vi "LabCode.vi"() -> ()   [LabVIEW 2020]
panel:
  in  "STOP":bool
  in  "GREEN":bool
  in  "YELLOW":bool
  in  "RED":bool
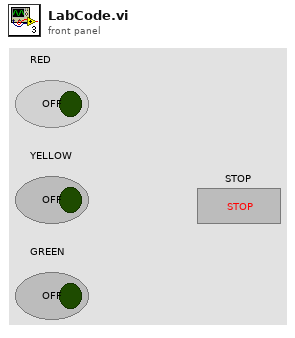
[diagram p1: front panel]
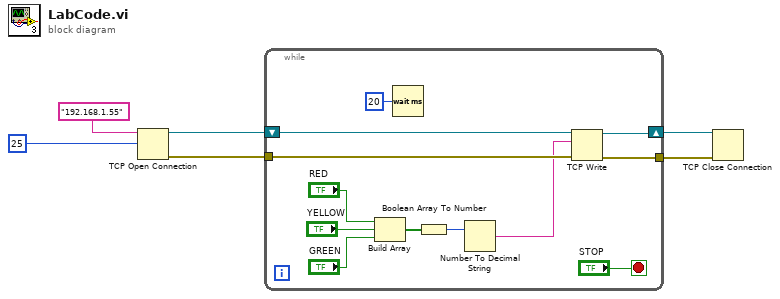
[diagram p0: block diagram]
diagram:
  n1 = TCP Open Connection(address="192.168.1.55", remote port or service name=u16 25) -> (connection ID=w4:refnum<k5>, error out=w3:errorcluster)  [unwired: 3 in]
  n2 = while {
    tunnel: w3 -> [w16]
    shift-right: [w15] -> w2
    shift-left: w4 -> [w17]
    tunnel: [w8] -> w1
    stop <- "STOP" stop-if-true
    n3 = Build Array("RED", "YELLOW", "GREEN") -> (w11:bool[])
    n4 = Wait (ms)(milliseconds to wait=u32 20) -> ()  [unwired: 1 out]
    n5 = Boolean Array To Number(Boolean array=w11) -> (number=w10:u32)
    n6 = Number To Decimal String(number=w10) -> (decimal integer string=w9:string)  [unwired: 1 in]
    n7 = TCP Write(connection ID=w17, data in=w9, error in (no error)=w16) -> (connection ID out=w15:refnum<k5>, error out=w8:errorcluster)  [unwired: 1 in, 1 out]
  }
  n8 = TCP Close Connection(connection ID=w2, error in (no error)=w1) -> ()  [unwired: 1 in, 2 out]
